vi "Dashboard Main.vi"() -> ()   [LabVIEW 2015]
uses:
  <vilib>/Utility/miscctls.llb/LVRowAndColumnTypeDef.ctl
  <vilib>/event_ctls.llb/eventvkey.ctl
  <vilib>/Rock Robotics/WPI/Dashboard/WPI_DashboardLogging Global.vi
  <vilib>/Utility/config.llb/Write Key (String).vi
  <vilib>/Utility/config.llb/Write Key (I32).vi
  <vilib>/Utility/config.llb/NI_LVConfig.lvlib
panel:
  in  "TCP":refnum<k5>
  in  "Rec Mode":enum32{"Stop", "Record", "Playback"}(radio)
  in  "Vision":u16(ring) items=["Camera Off", "USB Camera SW", "USB Camera HW", "IP Camera"]
  out "Camera IP":string
  out "Image Message":string="Timeout in Camera Communications"
  in  "Dashboard Tab":T1(tab)
  in  "Auto":string(combo)
  out "Velocity":dbl
  out "Can Hit":bool
  out "Visible Image":bool
  out "Can Hit":bool
  out "Possible Velocity":bool
  out "Centered":bool
  in  "Select Auto":string(combo)
  out "NT Connection":bool
  in  "Camera Settings":T2={"Frame Rate"=30, "Compression"=30, "Size"=1} {"Frame Rate" scale=1.0..30.0; "Size" items=["640x480", "320x240", "160x120"]}
  out "Mode":T3(ring)=enum."Auto Disabled"
  in  "DB Camera Config":bool
  out "fps":dbl format="%#.1g"
  out "Mbps":dbl format="%#.1g"
  out "Mbps LED":bool
  in  "DB/String 9":string
  in  "DB/String 8":string
  in  "DB/String 7":string
  in  "DB/String 6":string
  in  "DB/String 5":string
  in  "DB/String 4":string
  in  "DB/String 3":string
  in  "DB/String 2":string
  in  "DB/String 1":string
  in  "DB/String 0":string
  in  "DB/Slider 0":dbl(slide) scale=0.0..5.0
  in  "DB/Slider 1":dbl(slide) scale=0.0..5.0
  in  "DB/Slider 2":dbl(slide) scale=0.0..5.0
  in  "DB/Slider 3":dbl(slide) scale=0.0..5.0
  out "DB/LED 3":bool
  out "DB/LED 2":bool
  out "DB/LED 1":bool
  out "DB/LED 0":bool
  in  "DB/Button 3":bool
  in  "DB/Button 2":bool
  in  "DB/Button 1":bool
  in  "DB/Button 0":bool caption="New Name"
  in  "Test Slider":dbl(slide) scale=0.0..100.0 scale format="%#_3g"
  in  "On/Off":bool caption="Solenoid"
  in  "Test Name":u16(ring) items=["Select the test to run..."]
  in  "Test Tree":string(tree)
  in  "Motor":cluster{"Value":dbl, "Enable":bool} {"Value" scale=-1.0..1.0 scale format="%#_3g"}
  out "Progress":T4 {"Test Progress" scale=0.0..100.0}
  in  "Rev/Fwd":cluster{"Forward":bool, "Reverse":bool}
  in  "Test Ring":u16(ring) items=["Monochrome", "Color"]
  out "Cmd Status":string
  in  "Execute Command":bool
  in  "Command Params":string[][](table)
  in  "Command Selection":i32(listbox)
  in  "CheckList":i32(listbox)
  out "Tree":string(tree)
  out "Camera Image":T5(plugin-control)
  out "Background":bool
  # "This tab is a great place for autonomous settings and robot-specific values.\nPlace controls and indicators inside this tab and match name to\nDashboard Variables on robot. You can also delete this comment."
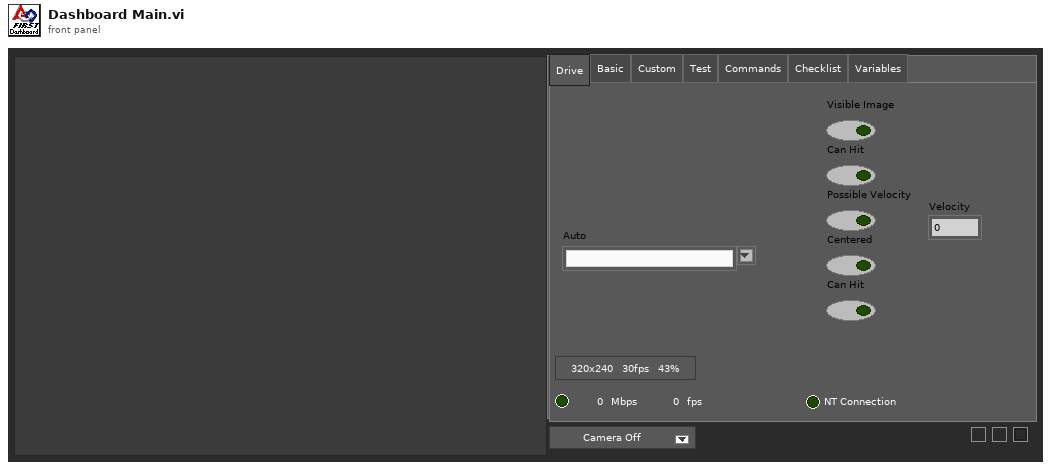
[diagram p1: front panel]
types:
  T1 = enum32{"Drive", "Basic", "Custom", "Test", "Commands", "Checklist", "Variables"}
  T2 = cluster{"Frame Rate":i32, "Compression":i32, "Size":u16}
  T3 = enum8{"Tele-Op Disabled", "Tele-Op Enabled", "Auto Disabled", "Auto Enabled", "Test Disabled", "Test Enabled", "Disconnected", "No Code", "E-Stop"}
  T4 = cluster{"Test Progress":u8, "Test Progress Text":string}
  T5 = typedef "IMAQ Image.ctl" = refnum<image>
  T6 = cluster{"IDs":cluster{"RPC field ID":u16, "Unique ID":u16}, "String":string}
  T7 = enum32{"Drive", "Basic", "Custom", "Test", "Checklist", "Variables"}
  T8 = typedef "Image Type" = u32
  T9 = cluster{"Camera Image":refnum<vi>, "Dashboard Tab":refnum<vi>, "Background":refnum<vi>, "Vision":refnum<vi>, "Rec Mode":refnum<vi>, "Test Slider":refnum<vi>, "On/Off ":refnum<vi>, "Test Ring":refnum<vi>, "Rev/Fwd":refnum<vi>, "Test Name":refnum<vi>, "Motor":refnum<vi>, "Progress":refnum<vi>, "CheckList":refnum<vi>, "Tree":refnum<vi>, "Test Tree":refnum<vi>, "Command Params":refnum<vi>, "Command Selection":refnum<vi>, "Execute Command":refnum<vi>, "Cmd Status":refnum<vi>}
  T10 = cluster{"Error Strings":string, "Disable Counts":cluster{u16, u16}, "Rail Faults":cluster{u16, u16, u16}, "Robot IP":string, "DB Mode":u8, "Event Info":cluster{"Name":string, "Type":u8, "Number":u16, "Replay":u8}, "Camera Addr":string}
  T11 = cluster{"Storage":cluster{"Disk Free":u64, "RAM Block":u32, "RAM free":u32}, "CPU Utilization":cluster{"CPU % ISR":sgl, "CPU % Time Crit":sgl, "CPU % Timed Str":sgl, "CPU % High":sgl, "CPU % Above":sgl, "CPU % Normal":sgl, "CPU % Low":sgl}, "CAN":cluster{"% Bus Utilization":sgl, "Bus Off Cnt":u32, "TX_FIFO Full Cnt":u32, "Receive Error Cnt":u8, "Transmit Error Cnt":u8}, "HID":cluster{"HID Outputs":u32, "Rumble Low":u16, "Rumble High":u16}[]}
  T12 = cluster{"Status bits":cluster{"Test Mode":bool, "Autonomous":bool, "Enabled":bool, "Code Start":bool, "Brownout":bool, "Reserved 2":bool, "Reserved 3":bool, "E-Stop":bool}, "Code Trace":cluster{"Disabled":bool, "TeleOp":bool, "Auto":bool, "Test":bool}, "Controller Type":enum16{"unknown", "cRIO", "roboRio"}, "Code?":enum16{"unknown", "noCode", "code"}, "Battery V":dbl}
  T13 = cluster{"Control Bits":cluster{"TestMode":bool, "Autonomous":bool, "Enabled":bool, "FMS Present":bool, bool, bool, bool, "E-Stop":bool}, "Team Station ":u8, "Countdown":sgl, "Joystick Values":cluster{"Axes":dbl[], "Buttons":bool[], "POVs":i16[]}[]}
  T14 = typedef "NI_LVConfig.lvlib/Config Data RefNum.ctl" = refnum<k1>
  T15 = cluster{"Operation":enum16{"Update", "Clear"}, "Color Box":u32}[]
  T16 = typedef "eventvkey.ctl" = enum16{"ASCII", "Enter", "Return", "Shift", "Ctrl", "Alt", "Cmd", "Opt", "Caps", "NumLock", "Clear", "Break", "Up", "Down", "Left", "Right", "Insert", "Delete", "Home", "End", "PageUp", "PageDown", "Escape", "Help", "Pause", "ScrollLock", "F1", "F2", "F3", "F4", "F5", "F6", "F7", "F8", "F9", "F10", "F11", "F12", "F13", "F14", "F15", "F16", "F17", "F18", "F19", "F20", "F21", "F22", "F23", "F24", "Play", "VolumeUp", "VolumeDown", "Mute", "Two Byte Char"}
  T17 = cluster{"Image Size":bool, "Image Type":bool, "Pixel Value":bool, "ROI Information":bool, "Zoom Factor":bool}
  T18 = enum8{"Enabled", "Disabled", "Disabled and Grayed Out"}
  T19 = cluster{"Operation":enum16{"Update", "Clear"}, "Color Box":u32}
  T20 = typedef "LVRowAndColumnTypeDef.ctl" = cluster{"Row":i32, "Column":i32}
  T21 = cluster{"Shift":bool, "Ctrl":bool, "Alt":bool, "Cmd":bool, "Opt":bool}
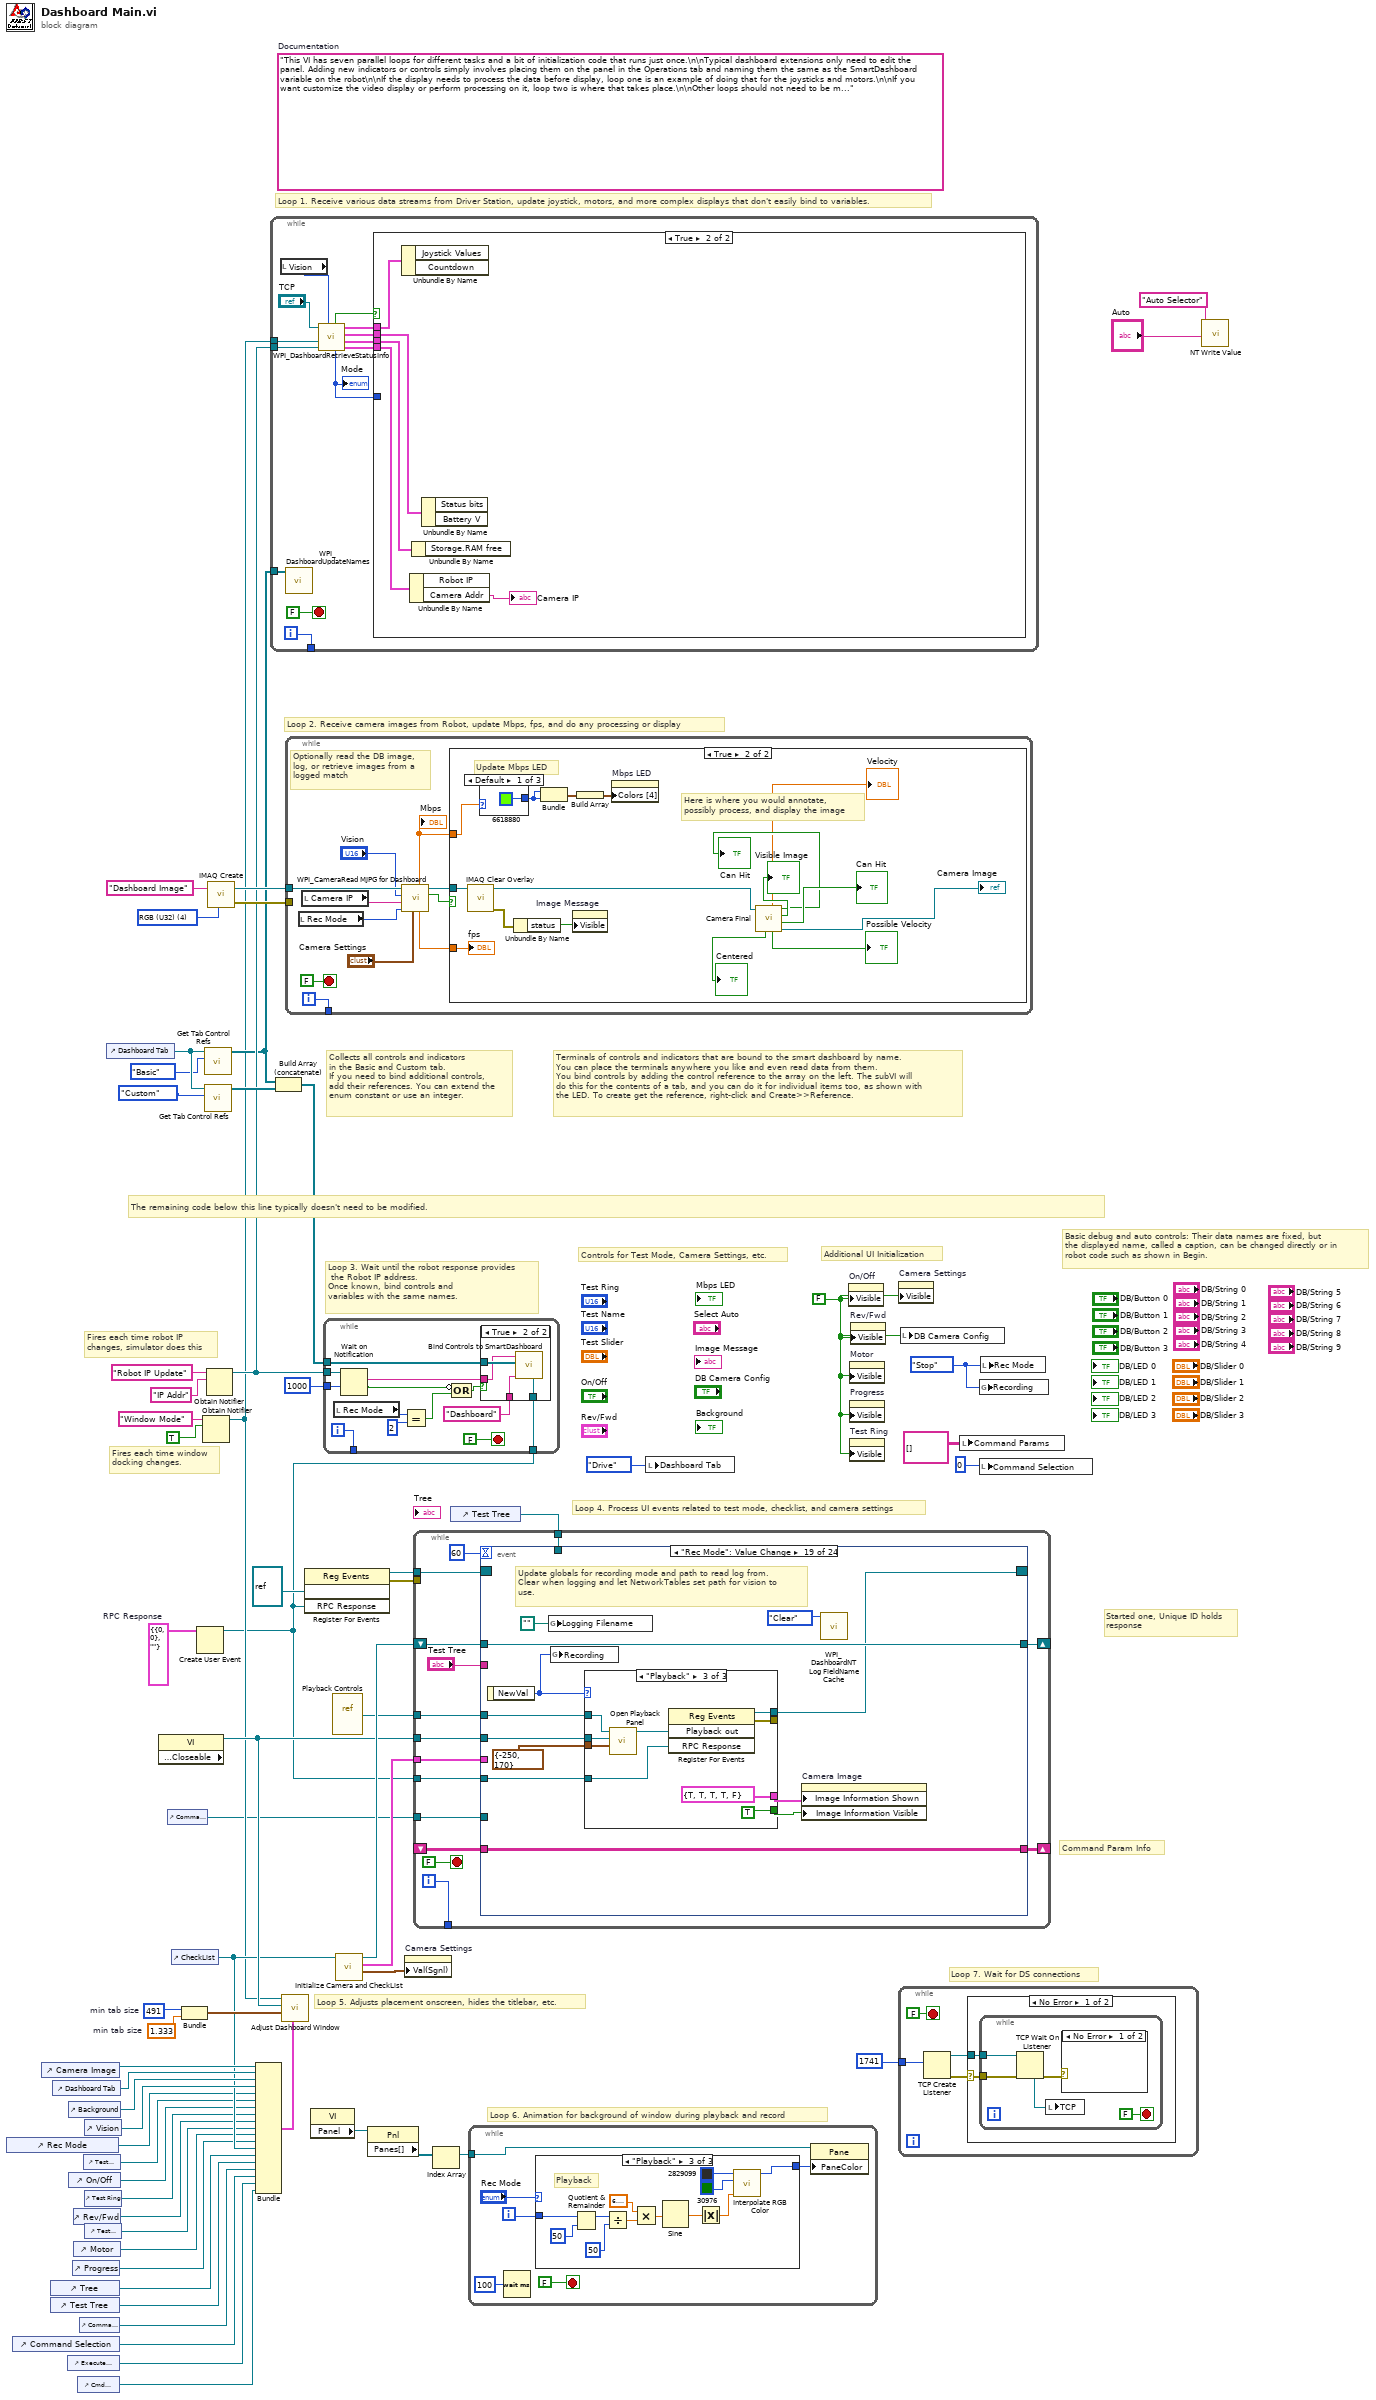
[diagram p0: block diagram]
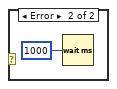
[diagram p2: hidden frame]
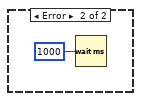
[diagram p3: hidden frame]
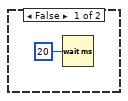
[diagram p4: hidden frame]
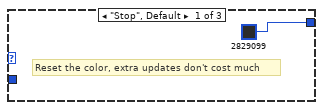
[diagram p5: hidden frame]
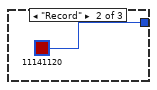
[diagram p6: hidden frame]
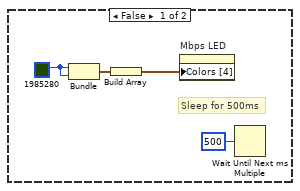
[diagram p8: hidden frame]
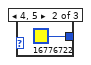
[diagram p9: hidden frame]
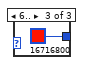
[diagram p10: hidden frame]
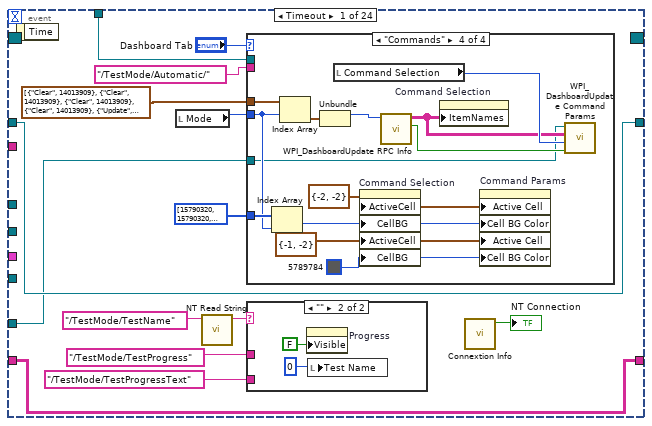
[diagram p11: hidden frame]
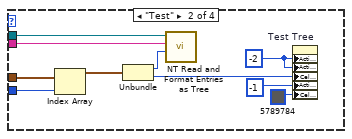
[diagram p13: hidden frame]
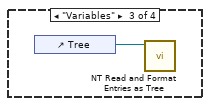
[diagram p14: hidden frame]
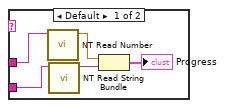
[diagram p15: hidden frame]
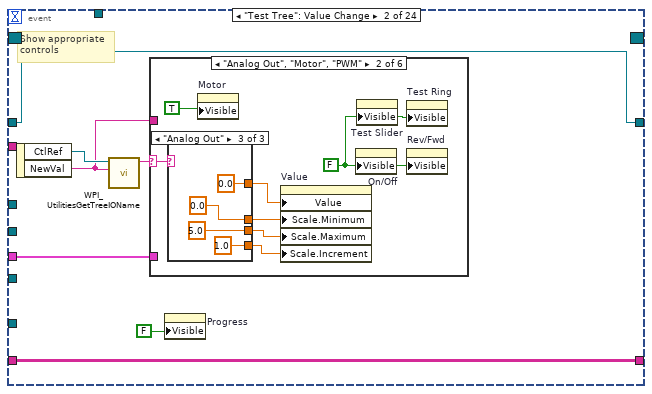
[diagram p16: hidden frame]
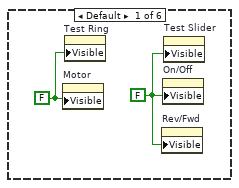
[diagram p17: hidden frame]
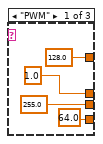
[diagram p18: hidden frame]
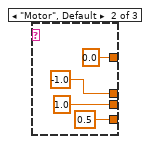
[diagram p19: hidden frame]
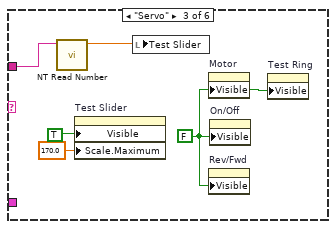
[diagram p20: hidden frame]
diagram:
  w9 = T6 {"IDs"={"RPC field ID"=0, "Unique ID"=0}, "String"=""}  # RPC Response
  w35 = 491  # min tab size
  w34 = 1.333  # min tab size
  w43 = enum32{"Stop", "Record", "Playback"}."Stop" ("Rec Mode")
  w17 = FALSE ("Visible")
  (unwired) "This VI has seven parallel loops for different tasks and a bit of initialization code that runs just once.\n\nTypical dashboard extensions only need to edit the panel. Adding new indicators or controls simply involves placing them on the panel in the Operations tab and naming them the same as the SmartDashboard variable on the robot\n\nIf the display needs to process the data before display, loop one is an example of doing that for the joysticks and motors.\n\nIf you want customize the video display or perform processing on it, loop two is where that takes place.\n\nOther loops should not need to be modified. They are pretty standard, and document the task they perform."  # Documentation
  w63 = T8 4 items=["Grayscale (U8)", "Grayscale (I16)", "Grayscale (SGL)", "Complex (CSG)", "RGB (U32)", "HSL (U32)", "RGB (U64)"] ("Image Type")
  # "Command Param Info"
  # "Started one, Unique ID holds\nresponse"
  # "Loop 7. Wait for DS connections"
  # "Basic debug and auto controls: Their data names are fixed, but\nthe displayed name, called a caption, can be changed directly or in\nrobot code such as shown in Begin."
  # "Controls for Test Mode, Camera Settings, etc."
  # "Additional UI Initialization"
  # "Loop 6. Animation for background of window during playback and record"
  # "Fires each time robot IP\nchanges, simulator does this"
  # "Fires each time window\ndocking changes."
  # "Collects all controls and indicators\nin the Basic and Custom tab.\nIf you need to bind additional controls,\nadd their references. You can extend the\nenum constant or use an integer."
  # "The remaining code below this line typically doesn't need to be modified."
  # "Loop 4. Process UI events related to test mode, checklist, and camera settings"
  # "Terminals of controls and indicators that are bound to the smart dashboard by name.\nYou can place the terminals anywhere you like and even read data from them.\nYou bind controls by adding the control reference to the array on the left. The subVI will\ndo this for the contents of a tab, and you can do it for individual items too, as shown with\nthe LED. To create get the reference, right-click and Create>>Reference."
  # "Loop 3. Wait until the robot response provides\n the Robot IP address.\nOnce known, bind controls and\nvariables with the same names."
  # "Loop 5. Adjusts placement onscreen, hides the titlebar, etc."
  # "Loop 1. Receive various data streams from Driver Station, update joystick, motors, and more complex displays that don't easily bind to variables."
  # "Loop 2. Receive camera images from Robot, update Mbps, fps, and do any processing or display"
  n1 = control-ref of="Rec Mode"() -> (w23:refnum<vi>)
  n2 = control-ref of="Command Selection"() -> (w8:refnum<vi>)
  n3 = control-ref of="Camera Image"() -> (w38:refnum<vi>)
  n4 = control-ref of="Tree"() -> (w27:refnum<vi>)
  n5 = control-ref of="Test Tree"() -> (w26:refnum<vi>)
  n6 = control-ref of="Dashboard Tab"() -> (w37:refnum<vi>)
  n7 = control-ref of="Execute Command"() -> (w10:refnum<vi>)
  n8 = control-ref of="Background"() -> (w32:refnum<vi>)
  n9 = control-ref of="On/Off"() -> (w21:refnum<vi>)
  n10 = control-ref of="Progress"() -> (w18:refnum<vi>)
  n11 = control-ref of="Rev/Fwd"() -> (w19:refnum<vi>)
  n12 = control-ref of="Motor"() -> (w24:refnum<vi>)
  n13 = control-ref of="Cmd Status"() -> (w4:refnum<vi>)
  n14 = control-ref of="Command Params"() -> (w11:refnum<vi>)
  n15 = control-ref of="Test Slider"() -> (w22:refnum<vi>)
  n16 = control-ref of="Vision"() -> (w36:refnum<vi>)
  n17 = control-ref of="Test Ring"() -> (w20:refnum<vi>)
  n18 = control-ref of="Test Name"() -> (w25:refnum<vi>)
  n19 = control-ref of="Dashboard Tab"() -> (w41:refnum<vi>)
  n20 = property class="VI" props=["Front Panel.Closeable"]() -> (reference out=w42:refnum<vi>)  [unwired: 2 in, 2 out]
  n21 = control-ref of="Command Params"() -> (w3:refnum<vi>)
  n22 = control-ref of="CheckList"() -> (w28:refnum<vi>)
  n23 = Bundle("min tab size"=w35, "min tab size"=w34) -> (w33:cluster{"min tab size":i32, "min tab size":dbl})  [unwired: 1 in]
  n24 = Create User Event(user event datatype=w9) -> (user event=w5:refnum<user-event>)  [unwired: 1 in, 1 out]
  n25 = Obtain Notifier(name (unnamed)="Window Mode", notification data type=TRUE) -> (notifier out=w14:refnum<notifier>)  [unwired: 2 in, 2 out]
  n26 = call <vilib>:"Get Tab Control Refs.vi"("Page Index"=T7."Basic" ("Dashboard Tab"), "TabControl in"=w41) -> ("ControlsOnPage"=w15:refnum<vi>[])  [unwired: 9 in]
  n27 = call <vilib>:"Get Tab Control Refs.vi"("Page Index"=T7."Custom" ("Dashboard Tab"), "TabControl in"=w41) -> ("ControlsOnPage"=w40:refnum<vi>[])  [unwired: 9 in]
  n28 = Obtain Notifier(name (unnamed)="Robot IP Update", notification data type="IP Addr" ("name (unnamed)")) -> (notifier out=w16:refnum<notifier>)  [unwired: 2 in, 2 out]
  n29 = call "IMAQ Create"("Image Name"="Dashboard Image", "Image Type"=w63) -> ("New Image"=w61:T5, "error out"=w60:errorcluster)  [unwired: 2 in, 1 out]
  n30 = Bundle("Camera Image"=w38, "Dashboard Tab"=w37, "Background"=w32, "Vision"=w36, "Rec Mode"=w23, "Test Slider"=w22, "On/Off"=w21, "Test Ring"=w20, "Rev/Fwd"=w19, "Test Name"=w25, "Motor"=w24, "Progress"=w18, "CheckList"=w28, "Tree"=w27, "Test Tree"=w26, "Command Params"=w11, "Command Selection"=w8, "Execute Command"=w10, "Cmd Status"=w4) -> (w29:T9)  [unwired: 1 in]
  n31 = while {
    tunnel: [w75] -> _
    tunnel: w16 -> [w69]
    tunnel: w15 -> [w68]
    tunnel: w14 -> [w64]
    i -> [w75]
    stop <- FALSE stop-if-true
    n32 = local read "Vision"() -> (w66:u16)
    n33 = call <vilib>:"WPI_DashboardUpdateNames.vi"("Controls on Tab"=w68) -> ()  [unwired: 11 in]
    n34 = call <vilib>:"WPI_DashboardRetrieveStatusInfo.vi"("Vision"=w66, "Binding Refnum"=w69, "Window Mode Notifier"=w64, "TCP Cnx"="TCP") -> ("Power and Errors"=w70:T10, "Robot Metrics"=w73:T11, "Status Info"=w74:T12, "Control Info"=w71:T13, "Robot Mode"=w67:T3, "Process?"=w72:bool)  [unwired: 2 in]
    "Mode" <- w67
    n35 = case shown="True" w72 {
      tunnel: w74 -> [_ w82]
      tunnel: w73 -> [_ w81]
      tunnel: w71 -> [_ w80]
      tunnel: w70 -> [_ w79]
      tunnel: w67 -> [_ _]
      frame False {
        n36 = Wait (ms)(milliseconds to wait=u32 20) -> ()  [unwired: 1 out]
      }
      frame True {
        n37 = Unbundle By Name(w80) -> ()  [unwired: 2 out]
        n38 = Unbundle By Name(w79) -> ("Camera Addr"=→"Camera IP":string)  [unwired: 1 out]
        n39 = Unbundle By Name(w81) -> ()  [unwired: 1 out]
        n40 = Unbundle By Name(w82) -> ()  [unwired: 2 out]
      }
    }
  }
  n41 = Build Array (concatenate)(w15, w40) -> (w39:refnum<vi>[])
  n42 = call "Adjust Dashboard Window.vi"("Sizing Refnums"=w29, "Size Constraints"=w33, "VI"=w42, "WIn Mode"=w14) -> ()  [unwired: 8 in]
  n43 = while {
    tunnel: w61 -> [w91]
    tunnel: w60 -> [_]
    tunnel: [w92] -> _
    i -> [w92]
    stop <- FALSE stop-if-true
    # "Optionally read the DB image,\nlog, or retrieve images from a\nlogged match"
    n44 = local read "Rec Mode"() -> (w86:enum32{"Stop", "Record", "Playback"})
    n45 = local read "Camera IP"() -> (w84:string)
    n46 = call <vilib>:"WPI_CameraRead MJPG for Dashboard.vi"("Camera Settings"="Camera Settings", "Rec Mode"=w86, "Camera IP"=w84, "Camera Mode"="Vision", "Refnum in"=w91) -> ("Active"=w89:bool, "Refnum out"=w90:T5, "FPS"=w88:dbl, "Bandwidth (Mbps)"=w83:dbl)  [unwired: 3 in]
    "Mbps" <- w83
    n47 = case shown="True" w89 {
      tunnel: w90 -> [_ w108]
      tunnel: w83 -> [_ w107]
      tunnel: w88 -> [_ w106]
      frame False {
        w94 = u32 1985280 ("Color Box")
        # "Sleep for 500ms"
        n48 = Bundle("Color Box"=w94, "Color Box"=w94) -> (w96:cluster{"Color Box":u32, "Color Box":u32})  [unwired: 1 out]
        n49 = Build Array(w96) -> (w95:cluster{"Color Box":u32, "Color Box":u32}[])
        n50 = property on="Mbps LED" class="Bool (strict)"("Colors [4]"=w95) -> ()  [unwired: 2 in, 2 out]
        n51 = Wait Until Next ms Multiple(millisecond multiple=u32 500) -> ()  [unwired: 1 out]
      }
      frame True {
        # "Here is where you would annotate,\npossibly process, and display the image"
        # "Update Mbps LED"
        n52 = call "IMAQ Clear Overlay"("Image"=w108) -> ("error out"=w112:errorcluster, "Image Out"=w105:T5)  [unwired: 2 in, 7 out]
        n53 = case shown="Default" w107 {
          tunnel: [u32 6618880 ("Color Box") u32 16776722 ("Color Box") u32 16716800 ("Color Box")] -> w109
          frame Default {
          }
          frame 4, 5 {
          }
          frame 6.. {
          }
        }
        n54 = Unbundle By Name(w112) -> ("status"=w113:bool)
        n55 = Bundle("Color Box"=w109, "Color Box"=w109) -> (w111:cluster{"Color Box":u32, "Color Box":u32})  [unwired: 1 out]
        n56 = property on="Image Message" class="Str"("Visible"=w113) -> ()  [unwired: 2 in, 2 out]
        n57 = Build Array(w111) -> (w110:cluster{"Color Box":u32, "Color Box":u32}[])
        n58 = property on="Mbps LED" class="Bool (strict)"("Colors [4]"=w110) -> ()  [unwired: 2 in, 2 out]
        n59 = call "Camera Final.vi"("Image Src"=w105) -> ("Image Dst Out 2"=→"Camera Image":T5, "Can Fit"=→"Can Hit":bool, "Viable Image"=→"Visible Image":bool, "Can Hit"=→"Can Hit":bool, "Possible Velocity"=→"Possible Velocity":bool, "Velocity"=→"Velocity":dbl, "Centered"=→"Centered":bool)  [unwired: 4 in]
        "fps" <- w106
      }
    }
  }
  n60 = register-events(refnum<vi> refnum, w5) -> (reference out=w47:refnum<event-registration>, error out=w46:errorcluster)  [unwired: 2 in]
  n61 = property class="VI"() -> ("Panel"=w50:refnum<vi>)  [unwired: 2 in, 2 out]
  n62 = while {
    tunnel: w39 -> [w129]
    tunnel: w16 -> [w127]
    tunnel: [w125] -> _
    tunnel: u32 1000 ("milliseconds to wait") -> [w124]
    tunnel: w5 -> [w117]
    i -> [w125]
    stop <- FALSE stop-if-true
    n63 = local read "Rec Mode"() -> (w120:enum32{"Stop", "Record", "Playback"})
    n64 = Wait on Notification(notifier=w127, timeout in ms (-1)=w124) -> (notification=w126:string, timed out?=w122:bool)  [unwired: 2 in, 2 out]
    n65 = Equal?(x=w120, y=u16 2 ("Rec Mode")) -> (x = y?=w121:bool)
    n66 = Compound Arithmetic op=OR(invert w122, w121) -> (w123:bool)
    n67 = case shown="True" w123 {
      tunnel: w129 -> [_ w133]
      tunnel: w126 -> [_ w132]
      tunnel: "Dashboard" -> [_ w131]
      tunnel: w117 -> [_ w130]
      frame False {
      }
      frame True {
        n68 = call <vilib>:"Bind Controls to SmartDashboard.vi"("RPC ref"=w130, "Client Name"=w131, "Bound Control Refs"=w133, "Server IP Address"=w132) -> ()  [unwired: 8 in]
      }
    }
  }
  n69 = vi-ref "Playback Controls.vi"() -> (w48:refnum<vi>)
  n70 = call "Initialize Camera and CheckList.vi"("ListBox in"=w28) -> ("Cluster"=w54:cluster{"value":i32, "value":i32, "index":i32}, "Array"=w55:cluster{string[]}[], "File Refnum"=w53:T14)  [unwired: 8 in]
  n71 = property class="Pnl"(reference=w50) -> ("Panes[]"=w51:refnum<vi>[])  [unwired: 1 in, 2 out]
  n72 = property on="Camera Settings" class="Clust (strict)"("Val(Sgnl)"=w54) -> ()  [unwired: 2 in, 2 out]
  n73 = Index Array(array=w51) -> (element=w49:refnum<vi>)  [unwired: 1 in]
  n74 = control-ref of="Test Tree"() -> (w52:refnum<vi>)
  n75 = while {
    tunnel: w55 -> [w145]
    shift-right: [w144] -> _
    shift-left: w53 -> [w143]
    tunnel: [w142] -> _
    tunnel: w52 -> [w141]
    tunnel: w48 -> [w140]
    tunnel: w47 -> [w139]
    tunnel: w46 -> [_]
    tunnel: w42 -> [w138]
    tunnel: w5 -> [w137]
    tunnel: w3 -> [w136]
    shift-right: [w135] -> _
    shift-left: _ -> [w134]
    i -> [w142]
    stop <- FALSE stop-if-true
    n76 = event shown="[18] \"Rec Mode\": Value Change" {
      selector: w139 -> [_ _ _ _ _ _ _ _ _ _ _ _ _ _ _ _ _ _ _ _ _ _ _ _]
      dyn-events: [_ _ _ _ _ _ _ _ _ _ _ _ _ _ _ _ _ _ w454 _ _ _ _ _] -> _
      timeout: u32 60 ("milliseconds to wait") -> [_ _ _ _ _ _ _ _ _ _ _ _ _ _ _ _ _ _ _ _ _ _ _ _]
      tunnel: w141 -> [w159 _ _ _ _ _ _ _ _ _ _ _ _ _ _ _ _ _ _ _ _ _ _ _]
      tunnel: "Test Tree" -> [_ _ _ _ _ _ _ _ _ _ _ _ _ w417 w426 w429 w434 w443 _ _ _ _ _ _]
      tunnel: w145 -> [_ w196 _ _ _ _ _ _ _ _ _ w379 w410 _ _ _ _ _ _ _ _ _ _ _]
      tunnel: [w156 w195 w299 w305 w315 w319 w325 w337 w345 w351 w364 w378 w403 w416 w424 w428 w433 w442 w456 w472 w474 w482 w493 w498] -> w144
      tunnel: w143 -> [w156 w195 w299 w305 w315 w319 w325 w337 w345 w351 w364 w377 w403 w416 w424 w428 w433 w442 w456 w472 w474 w482 w493 w498]
      tunnel: w140 -> [_ _ _ _ _ _ _ _ _ _ _ _ _ _ _ _ _ _ w457 _ w477 _ _ _]
      tunnel: w138 -> [_ _ _ _ _ _ _ _ _ _ _ _ _ _ _ _ _ _ w452 _ _ _ _ _]
      tunnel: w137 -> [_ _ _ _ _ _ _ _ _ _ _ _ _ _ _ _ _ _ w448 _ _ _ _ _]
      tunnel: w136 -> [w151 _ _ _ _ _ w323 _ _ _ _ _ _ _ _ _ _ _ _ _ _ _ _ _]
      tunnel: [w150 w194 w298 w304 w314 w320 w321 w331 w342 w350 w363 w376 w402 w415 w423 w427 w432 w441 w447 w470 w473 w478 w486 w499] -> w135
      tunnel: w134 -> [w150 w194 w298 w304 w314 w320 w321 _ _ w350 w363 w376 w402 w415 w423 w427 w432 w441 w447 w470 w473 w478 w486 w499]
      event Timeout {
        n77 = event-data() -> ()  [unwired: 1 in, 1 out]
        n78 = local read "Mode"() -> (w153:T3)
        n79 = call <vilib>:"NT Read String.vi"("Name"="/TestMode/TestName") -> ("String"=w161:string)  [unwired: 9 in, 1 out]
        n80 = case shown="\"Commands\"" "Dashboard Tab" {
          tunnel: w159 -> [_ w172 _ _]
          tunnel: "/TestMode/Automatic/" ("Name Pattern") -> [_ w171 _ _]
          tunnel: T15 [{"Operation"=enum."Clear", "Color Box"=14013909}, {"Operation"=enum."Clear", "Color Box"=14013909}, {"Operation"=enum."Clear", "Color Box"=14013909}, {"Operation"=enum."Clear", "Color Box"=14013909}, {"Operation"=enum."Update", "Color Box"=14013909}, {"Operation"=enum."Update", "Color Box"=16777215}, {"Operation"=enum."Clear", "Color Box"=14013909}, {"Operation"=enum."Clear", "Color Box"=14013909}, {"Operation"=enum."Clear", "Color Box"=14013909}] -> [_ w164 _ w181]
          tunnel: w153 -> [_ w163 _ w180]
          tunnel: u32[] [15790320, 15790320, 15790320, 15790320, 16777215, 16777215, 15790320, 15790320, 15790320] -> [_ _ _ w186]
          tunnel: w151 -> [_ _ _ w174]
          frame "Custom", Default {
          }
          frame "Test" {
            w170 = -2 ("Active Item:Row Number")
            n81 = Index Array(array=w164, index=w163) -> (element=w165:T19)
            n82 = Unbundle(w165) -> ("Operation"=w166:enum16{"Update", "Clear"}, "Color Box"=w167:u32)
            n83 = call <vilib>:"NT Read and Format Entries as Tree.vi"("Operation"=w166, "Name Pattern"=w171, "Tree Refnum"=w172) -> ()  [unwired: 7 in, 2 out]
            n84 = property on="Test Tree" class="Tree (strict)"("Active Item Row Number"=w170, "ActiveColNum"=w170, "CellBG"=w167, "Active Item Row Number"=-1 ("Active Item:Row Number"), "CellBG"=u32 5789784 ("Color Box")) -> ()  [unwired: 2 in, 2 out]
          }
          frame "Variables" {
            n85 = control-ref of="Tree"() -> (w173:refnum<vi>)
            n86 = call <vilib>:"NT Read and Format Entries as Tree.vi"("Tree Refnum"=w173) -> ()  [unwired: 9 in, 2 out]
          }
          frame "Commands" {
            w182 = u32 5789784 ("Color Box")
            w183 = T20 {"Row"=-1, "Column"=-2} ("Active Cell:Active Cell")
            w185 = T20 {"Row"=-2, "Column"=-2} ("Active Cell:Active Cell")
            n87 = Index Array(array=w186, index=w180) -> (element=w184:u32)
            n88 = Index Array(array=w181, index=w180) -> (element=w179:T19)
            n89 = Unbundle(w179) -> ("Operation"=w178:enum16{"Update", "Clear"})  [unwired: 1 out]
            n90 = local read "Command Selection"() -> (w177:i32)
            n91 = property on="Command Selection" class="MCListbox (strict)"("ActiveCell"=w185, "CellBG"=w184, "ActiveCell"=w183, "CellBG"=w182) -> ()  [unwired: 2 in, 2 out]
            n92 = call <vilib>:"WPI_DashboardUpdate RPC Info.vi"("Operation"=w178) -> ("update"=w176:bool, "commands"=w175:string[][])  [unwired: 9 in]
            n93 = property on="Command Selection" class="MCListbox (strict)"("ItemNames"=w175) -> ()  [unwired: 2 in, 2 out]
            n94 = property on="Command Params" class="Tbl (strict)"("Active Cell"=w185, "Cell BG Color"=w184, "Active Cell"=w183, "Cell BG Color"=w182) -> ()  [unwired: 2 in, 2 out]
            n95 = call <vilib>:"WPI_DashboardUpdate Command Params.vi"("Update"=w176, "NewVal"=w177, "Commands"=w175, "Param Tbl"=w174) -> ()  [unwired: 7 in, 1 out]
          }
        }
        n96 = case shown="\"\"" w161 {
          tunnel: "/TestMode/TestProgress" ("Name") -> [w188 _]
          tunnel: "/TestMode/TestProgressText" ("Name") -> [w187 _]
          frame Default {
            n97 = call <vilib>:"NT Read Number.vi"("Name"=w188) -> ("Numeric"=w189:dbl)  [unwired: 9 in, 1 out]
            n98 = call <vilib>:"NT Read String.vi"("Name"=w187) -> ("String"=w190:string)  [unwired: 9 in, 1 out]
            n99 = Bundle("Numeric"=w189, "String"=w190) -> (→"Progress":cluster{"Numeric":dbl, "String":string})  [unwired: 1 in]
          }
          frame "" {
            n100 = property on="Progress" class="Clust (strict)"("Visible"=FALSE) -> ()  [unwired: 2 in, 2 out]
            n101 = local write "Test Name"(u16 0) -> ()
          }
        }
        n102 = call <vilib>:"Connextion Info.vi"() -> ("Connected"=→"NT Connection":bool)  [unwired: 10 in, 1 out]
      }
      event "Test Tree": Value Change {
        # "Show appropriate\ncontrols"
        n103 = event-data() -> ("CtlRef"=w199:refnum<vi>, "NewVal"=w197:string)  [unwired: 1 in]
        n104 = call <vilib>:"WPI_UtilitiesGetTreeIOName.vi"("NewVal"=w197, "TreeControl in"=w199) -> ("I/O Name"=w200:string)  [unwired: 9 in]
        n105 = case shown="\"Analog Out\", \"Motor\", \"PWM\"" w200 {
          selector: w200 -> [_ w207 _ w229 w238 _]
          tunnel: w197 -> [_ _ w226 w228 _ w245]
          tunnel: w196 -> [_ _ _ _ _ w244]
          frame Default {
            w202 = FALSE ("Visible")
            w201 = FALSE ("Visible")
            n106 = property on="Motor" class="Clust (strict)"("Visible"=w201) -> ()  [unwired: 2 in, 2 out]
            n107 = property on="Test Ring" class="Ring (strict)"("Visible"=w201) -> ()  [unwired: 2 in, 2 out]
            n108 = property on="Rev/Fwd" class="Clust (strict)"("Visible"=w202) -> ()  [unwired: 2 in, 2 out]
            n109 = property on="On/Off" class="Bool (strict)"("Visible"=w202) -> ()  [unwired: 2 in, 2 out]
            n110 = property on="Test Slider" class="Slide (strict)"("Visible"=w202) -> ()  [unwired: 2 in, 2 out]
          }
          frame "Analog Out", "Motor", "PWM" {
            w208 = FALSE ("Visible")
            n111 = case shown="\"Analog Out\"" w207 {
              tunnel: [1.0 ("Value") -1.0 ("Value") 0.0 ("Value")] -> w206
              tunnel: [255.0 ("Value") 1.0 ("Value") 5.0 ("Value")] -> w205
              tunnel: [128.0 ("Value") 0.0 ("Value") 0.0 ("Value")] -> w204
              tunnel: [64.0 ("Value") 0.5 ("Value") 1.0 ("Value")] -> w203
              frame "PWM" {
              }
              frame "Motor", Default {
              }
              frame "Analog Out" {
              }
            }
            n112 = property on="Motor" class="Clust (strict)"("Visible"=TRUE) -> ()  [unwired: 2 in, 2 out]
            n113 = property on="Value" class="Slide (strict)"("Value"=w204, "Scale.Minimum"=w206, "Scale.Maximum"=w205, "Scale.Increment"=w203) -> ()  [unwired: 2 in, 2 out]
            n114 = property on="On/Off" class="Bool (strict)"("Visible"=w208) -> ()  [unwired: 2 in, 2 out]
            n115 = property on="Test Slider" class="Slide (strict)"("Visible"=w208) -> ()  [unwired: 2 in, 2 out]
            n116 = property on="Test Ring" class="Ring (strict)"("Visible"=w208) -> ()  [unwired: 2 in, 2 out]
            n117 = property on="Rev/Fwd" class="Clust (strict)"("Visible"=w208) -> ()  [unwired: 2 in, 2 out]
          }
          frame "Servo" {
            w224 = FALSE ("Visible")
            n118 = call <vilib>:"NT Read Number.vi"("Name"=w226) -> ("Numeric"=w225:dbl)  [unwired: 9 in, 1 out]
            n119 = property on="Test Slider" class="Slide (strict)"("Visible"=TRUE, "Scale.Maximum"=170.0 ("Scale.Range:Maximum")) -> ()  [unwired: 2 in, 2 out]
            n120 = local write "Test Slider"(w225) -> ()
            n121 = property on="Motor" class="Clust (strict)"("Visible"=w224) -> ()  [unwired: 2 in, 2 out]
            n122 = property on="Rev/Fwd" class="Clust (strict)"("Visible"=w224) -> ()  [unwired: 2 in, 2 out]
            n123 = property on="On/Off" class="Bool (strict)"("Visible"=w224) -> ()  [unwired: 2 in, 2 out]
            n124 = property on="Test Ring" class="Ring (strict)"("Visible"=w224) -> ()  [unwired: 2 in, 2 out]
          }
          frame "Relay", "Solenoid" {
            w227 = FALSE ("Visible")
            n125 = property on="Motor" class="Clust (strict)"("Visible"=w227) -> ()  [unwired: 2 in, 2 out]
            n126 = property on="Test Slider" class="Slide (strict)"("Visible"=w227) -> ()  [unwired: 2 in, 2 out]
            n127 = Search and Replace String(input string=w228, search string="/Value  **", replace string="/Direction") -> (result string=w234:string)  [unwired: 5 in, 3 out]
            n128 = property on="Test Ring" class="Ring (strict)"("Visible"=w227) -> ()  [unwired: 2 in, 2 out]
            n129 = call <vilib>:"NT Read String.vi"("Name"=w234) -> ("String"=w232:string)  [unwired: 9 in, 1 out]
            n130 = Equal?(x="Both directions", y=w232) -> (x = y?=w230:bool)
            n131 = Not(x=w230) -> (.not. x?=w231:bool)
            n132 = property on="Rev/Fwd" class="Clust (strict)"("Visible"=w230) -> ()  [unwired: 2 in, 2 out]
            n133 = property on="On/Off" class="Bool (strict)"("Visible"=w231, "Caption.Text"=w229) -> ()  [unwired: 2 in, 2 out]
          }
          frame "Compressor", "Digital Out" {
            w237 = FALSE ("Visible")
            # "Get direction and finish"
            n134 = property on="Motor" class="Clust (strict)"("Visible"=w237) -> ()  [unwired: 2 in, 2 out]
            n135 = property on="Test Slider" class="Slide (strict)"("Visible"=w237) -> ()  [unwired: 2 in, 2 out]
            n136 = property on="Test Ring" class="Ring (strict)"("Visible"=w237) -> ()  [unwired: 2 in, 2 out]
            n137 = property on="On/Off" class="Bool (strict)"("Visible"=TRUE, "Caption.Text"=w238) -> ()  [unwired: 2 in, 2 out]
            n138 = property on="Rev/Fwd" class="Clust (strict)"("Visible"=FALSE) -> ()  [unwired: 2 in, 2 out]
          }
          frame "Camera" {
            n139 = call <vilib>:"Get Last Path Segment.vi"("String in"=w245) -> ("String out"=w246:string)  [unwired: 10 in]
            n140 = property on="On/Off" class="Bool (strict)"("Visible"=FALSE) -> ()  [unwired: 2 in, 2 out]
            n141 = property on="Motor" class="Clust (strict)"("Visible"=FALSE) -> ()  [unwired: 2 in, 2 out]
            n142 = property on="Rev/Fwd" class="Clust (strict)"("Visible"=FALSE) -> ()  [unwired: 2 in, 2 out]
            n143 = case shown="\"White Balance  **\"" w246 {
              tunnel: w245 -> [w252 w261 w270 w279 w288 _ w294]
              tunnel: w244 -> [w250 w258 w267 w276 w285 _ _]
              frame "Size  **" {
                n144 = Index Array(array=w250) -> (element=w249:cluster{string[]})  [unwired: 1 in]
                n145 = call <vilib>:"NT Read String.vi"("Name"=w252) -> ("String"=w251:string)  [unwired: 9 in, 1 out]
                n146 = Unbundle(w249) -> (w247:string[])
                n147 = Match First String(2:w247, 3:w251) -> (0:w248:i32)  [unwired: 1 out]
                n148 = property on="Test Ring" class="Ring (strict)"("Value"=w248, "Strings []"=w247) -> ()  [unwired: 2 in, 2 out]
                n149 = property on="Test Ring" class="Ring (strict)"("Visible"=TRUE) -> ()  [unwired: 2 in, 2 out]
                n150 = property on="Test Slider" class="Slide (strict)"("Visible"=FALSE) -> ()  [unwired: 2 in, 2 out]
              }
              frame "White Balance  **" {
                n151 = Index Array(array=w258, index=1) -> (element=w259:cluster{string[]})
                n152 = call <vilib>:"NT Read String.vi"("Name"=w261) -> ("String"=w260:string)  [unwired: 9 in, 1 out]
                n153 = Unbundle(w259) -> (w256:string[])
                n154 = Match First String(2:w256, 3:w260) -> (0:w255:i32)  [unwired: 1 out]
                n155 = property on="Test Ring" class="Ring (strict)"("Value"=w255, "Strings []"=w256) -> ()  [unwired: 2 in, 2 out]
                n156 = property on="Test Ring" class="Ring (strict)"("Visible"=TRUE) -> ()  [unwired: 2 in, 2 out]
                n157 = property on="Test Slider" class="Slide (strict)"("Visible"=FALSE) -> ()  [unwired: 2 in, 2 out]
              }
              frame "Exposure  **" {
                n158 = Index Array(array=w267, index=2) -> (element=w268:cluster{string[]})
                n159 = call <vilib>:"NT Read String.vi"("Name"=w270) -> ("String"=w269:string)  [unwired: 9 in, 1 out]
                n160 = Unbundle(w268) -> (w264:string[])
                n161 = Match First String(2:w264, 3:w269) -> (0:w265:i32)  [unwired: 1 out]
                n162 = property on="Test Ring" class="Ring (strict)"("Value"=w265, "Strings []"=w264) -> ()  [unwired: 2 in, 2 out]
                n163 = property on="Test Ring" class="Ring (strict)"("Visible"=TRUE) -> ()  [unwired: 2 in, 2 out]
                n164 = property on="Test Slider" class="Slide (strict)"("Visible"=FALSE) -> ()  [unwired: 2 in, 2 out]
              }
              frame "Exposure Priority  **" {
                n165 = Index Array(array=w276, index=3) -> (element=w277:cluster{string[]})
                n166 = call <vilib>:"NT Read String.vi"("Name"=w279) -> ("String"=w278:string)  [unwired: 9 in, 1 out]
                n167 = Unbundle(w277) -> (w273:string[])
                n168 = Match First String(2:w273, 3:w278) -> (0:w274:i32)  [unwired: 1 out]
                n169 = property on="Test Ring" class="Ring (strict)"("Value"=w274, "Strings []"=w273) -> ()  [unwired: 2 in, 2 out]
                n170 = property on="Test Ring" class="Ring (strict)"("Visible"=TRUE) -> ()  [unwired: 2 in, 2 out]
                n171 = property on="Test Slider" class="Slide (strict)"("Visible"=FALSE) -> ()  [unwired: 2 in, 2 out]
              }
              frame "Color Enable  **" {
                n172 = Index Array(array=w285, index=4) -> (element=w286:cluster{string[]})
                n173 = call <vilib>:"NT Read String.vi"("Name"=w288) -> ("String"=w287:string)  [unwired: 9 in, 1 out]
                n174 = Unbundle(w286) -> (w282:string[])
                n175 = Match First String(2:w282, 3:w287) -> (0:w283:i32)  [unwired: 1 out]
                n176 = property on="Test Ring" class="Ring (strict)"("Value"=w283, "Strings []"=w282) -> ()  [unwired: 2 in, 2 out]
                n177 = property on="Test Ring" class="Ring (strict)"("Visible"=TRUE) -> ()  [unwired: 2 in, 2 out]
                n178 = property on="Test Slider" class="Slide (strict)"("Visible"=FALSE) -> ()  [unwired: 2 in, 2 out]
              }
              frame Default {
                n179 = property on="Test Ring" class="Ring (strict)"("Visible"=FALSE) -> ()  [unwired: 2 in, 2 out]
                n180 = property on="Test Slider" class="Slide (strict)"("Visible"=FALSE) -> ()  [unwired: 2 in, 2 out]
              }
              frame "Brightness  **", "Color Level  **", "Compression  **", "FPS  **", "Sharpness  **" {
                n181 = call <vilib>:"NT Read Number.vi"("Name"=w294) -> ("Numeric"=w293:dbl)  [unwired: 9 in, 1 out]
                n182 = local write "Test Slider"(w293) -> ()
                n183 = property on="Test Slider" class="Slide (strict)"("Visible"=TRUE, "Scale.Maximum"=100.0 ("Scale.Range:Maximum")) -> ()  [unwired: 2 in, 2 out]
                n184 = property on="Test Ring" class="Ring (strict)"("Visible"=FALSE) -> ()  [unwired: 2 in, 2 out]
              }
            }
          }
        }
        n185 = property on="Progress" class="Clust (strict)"("Visible"=FALSE) -> ()  [unwired: 2 in, 2 out]
      }
      event "Test Name": Mouse Enter {
        # "Populate the ring with the list of tests"
        n186 = event-data() -> ()  [unwired: 1 in, 1 out]
        n187 = call <vilib>:"NT Read String Array.vi"("Name"="/TestMode/TestList") -> ("String Array"=w303:string[])  [unwired: 9 in, 1 out]
        n188 = Build Array (concatenate)("Select the test to run...", w303) -> (w302:string[])
        n189 = property on="Test Name" class="Ring (strict)"("Strings []"=w302) -> ()  [unwired: 2 in, 2 out]
      }
      event "Test Name": Value Change {
        w306 = FALSE ("Visible")
        # "Tell the robot the test name to run"
        n190 = event-data() -> ("NewVal"=w310:u16)  [unwired: 1 in]
        n191 = property on="Test Name" class="Ring (strict)"() -> ("Strings []"=w311:string[])  [unwired: 2 in, 2 out]
        n192 = local write "Progress"(T4 {"Test Progress"=0, "Test Progress Text"=""} ("Progress")) -> ()
        n193 = Index Array(array=w311, index=w310) -> (element=w309:string)
        n194 = call <vilib>:"NT Write String.vi"("String"=w309, "Name"="/TestMode/TestName") -> ()  [unwired: 9 in, 1 out]
        n195 = property on="Progress" class="Clust (strict)"("Visible"=TRUE) -> ()  [unwired: 2 in, 2 out]
        n196 = property on="Motor" class="Clust (strict)"("Visible"=w306) -> ()  [unwired: 2 in, 2 out]
        n197 = property on="Test Slider" class="Slide (strict)"("Visible"=w306) -> ()  [unwired: 2 in, 2 out]
        n198 = property on="On/Off" class="Bool (strict)"("Visible"=w306) -> ()  [unwired: 2 in, 2 out]
        n199 = property on="Rev/Fwd" class="Clust (strict)"("Visible"=w306) -> ()  [unwired: 2 in, 2 out]
        n200 = property on="Test Ring" class="Ring (strict)"("Visible"=w306) -> ()  [unwired: 2 in, 2 out]
      }
      event "Select Auto": Mouse Enter {
        # "Populate the combo box with the list of autonomous options"
        n201 = event-data() -> ()  [unwired: 1 in, 1 out]
        n202 = call <vilib>:"NT Read String Array.vi"("Name"="Auto List") -> ("String Array"=w313:string[])  [unwired: 9 in, 1 out]
        n203 = property on="Select Auto" class="CmbBox"("Strings[]"=w313) -> ()  [unwired: 2 in, 2 out]
      }
      event "Select Auto": Value Change {
        # "User modified the Auto Selection. Write to NT variable so robot knows."
        n204 = event-data() -> ("NewVal"=w317:string)  [unwired: 1 in]
        n205 = call <vilib>:"NT Write String.vi"("String"=w317, "Name"="Auto Selector") -> ()  [unwired: 9 in, 1 out]
      }
      event "Command Selection": Value Change {
        # "Get the params and show in table"
        n206 = event-data() -> ("NewVal"=w324:i32)  [unwired: 1 in]
        n207 = property on="Command Selection" class="MCListbox (strict)"() -> ("ItemNames"=w322:string[][])  [unwired: 2 in, 2 out]
        n208 = call <vilib>:"WPI_DashboardUpdate Command Params.vi"("NewVal"=w324, "Commands"=w322, "Param Tbl"=w323) -> ()  [unwired: 8 in, 1 out]
      }
      event "Execute Command": Value Change {
        # "Started one, Unique ID holds\nresponse"
        n209 = event-data() -> ()  [unwired: 1 in, 1 out]
        n210 = property on="Command Selection" class="MCListbox (strict)"() -> ("ItemNames"=w336:string[][])  [unwired: 2 in, 2 out]
        n211 = Index Array(array=w336, index (row)="Command Selection", index (col)=0) -> (element=w334:string)
        n212 = call <vilib>:"Invoke Commands.vi"("Command Params"="Command Params", "Function Name"=w334) -> ("Params"=w330:u8, "Started"=w329:bool)  [unwired: 7 in, 1 out]
        n213 = Array Subset(array="Command Params", length (row)=w330) -> (w331:string[][])  [unwired: 3 in]
        n214 = Select(t="Executing" ("Cmd Status"), s=w329, f="" ("Cmd Status")) -> (s? t:f=→"Cmd Status":string)
      }
      event "Command Selection": Double Click {
        n215 = event-data() -> ("Row"=w346:i32)  [unwired: 1 in]
        n216 = property on="Command Selection" class="MCListbox (strict)"() -> ("ItemNames"=w349:string[][])  [unwired: 2 in, 2 out]
        n217 = local read "Command Params"() -> (w344:string[][])
        n218 = Index Array(array=w349, index (row)=w346, index (col)=0) -> (element=w347:string)
        n219 = call <vilib>:"Invoke Commands.vi"("Command Params"=w344, "Function Name"=w347) -> ("Params"=w343:u8, "Started"=w338:bool)  [unwired: 7 in, 1 out]
        n220 = Array Subset(array=w344, length (row)=w343) -> (w342:string[][])  [unwired: 3 in]
        n221 = Select(t="Executing" ("Cmd Status"), s=w338, f="" ("Cmd Status")) -> (s? t:f=w339:string)
        n222 = local write "Cmd Status"(w339) -> ()
      }
      event "CheckList": Double Click {
        # "Shift clears all"
        # "Update symbols on the listbox"
        n223 = event-data() -> ("PlatMods.Shift"=w352:bool, "Row"=w354:i32)  [unwired: 1 in]
        n224 = case shown="True" w352 {
          tunnel: w354 -> [w358 _]
          tunnel: 1 -> [w357 _]
          frame False {
            n225 = property on="CheckList" class="LstBox (strict)"() -> ("Item Symbols"=w356:i32[])  [unwired: 2 in, 2 out]
            n226 = Replace Array Subset(array=w356, new element=w357, index=w358) -> (w355:i32[])
            n227 = property on="CheckList" class="LstBox (strict)"("Item Symbols"=w355) -> ()  [unwired: 2 in, 2 out]
          }
          frame True {
            w359 = 0 ("Top Row")
            n228 = property on="CheckList" class="LstBox (strict)"() -> ("Number of Rows"=w361:u32)  [unwired: 2 in, 2 out]
            n229 = Initialize Array(0, w361) -> (w360:i32[])
            n230 = property on="CheckList" class="LstBox (strict)"("Top Row"=w359, "Value"=w359, "Item Symbols"=w360) -> ()  [unwired: 2 in, 2 out]
          }
        }
      }
      event "CheckList": Key Down {
        # "Update symbols on the listbox\nLeft and right keys check and uncheck"
        n231 = event-data() -> ("VKey"=w366:T16)  [unwired: 1 in]
        n232 = case shown="\"Left\", \"Right\"" w366 {
          selector: w366 -> [w371 _]
          tunnel: eventvkey."Left" ("VKey") -> [w369 _]
          frame "Left", "Right" {
            n233 = Equal?(x=w369, y=w371) -> (x = y?=w370:bool)
            n234 = Select(t=0, s=w370, f=1) -> (s? t:f=w372:i32)
            n235 = property on="CheckList" class="LstBox (strict)"() -> ("Item Symbols"=w375:i32[])  [unwired: 2 in, 2 out]
            n236 = Replace Array Subset(array=w375, new element=w372, index="CheckList") -> (w374:i32[])
            n237 = property on="CheckList" class="LstBox (strict)"("Item Symbols"=w374) -> ()  [unwired: 2 in, 2 out]
          }
          frame Default {
          }
        }
      }
      event "DB Camera Config": Value Change {
        # "Show or hide the cluster of controls, store in ini file"
        n238 = event-data() -> ("NewVal"=w380:bool)  [unwired: 1 in]
        n239 = case shown="False" w380 {
          tunnel: w379 -> [w389 _]
          tunnel: [w382 w400] -> w378
          tunnel: w377 -> [w381 w400]
          frame False {
            w396 = "Camera"
            w399 = FALSE ("Visible")
            n240 = local read "Camera Settings"() -> (w388:T2)
            n241 = Index Array(array=w389) -> (element=w392:cluster{string[]})  [unwired: 1 in]
            n242 = Unbundle(w388) -> ("Frame Rate"=w387:i32, "Compression"=w386:i32, "Size"=w390:u16)
            n243 = Unbundle(w392) -> (w391:string[])
            n244 = Index Array(array=w391, index=w390) -> (element=w385:string)
            n245 = call-poly <vilib>:"Write Key.vi"("section"=w396, "value"=w385, "key"="Size", "refnum"=w381) -> ("refnum out"=w398:T14)  [unwired: 2 in, 5 out]
            n246 = call-poly <vilib>:"Write Key.vi"("section"=w396, "value"=w387, "key"="FrameRate", "refnum"=w398) -> ("refnum out"=w397:T14)  [unwired: 1 in, 6 out]
            n247 = property on="Camera Settings" class="Clust (strict)"("Visible"=w399) -> ()  [unwired: 2 in, 2 out]
            n248 = local write "DB Camera Config"(w399) -> ()
            n249 = call-poly <vilib>:"Write Key.vi"("section"=w396, "value"=w386, "key"="Compression", "refnum"=w397) -> ("refnum out"=w383:T14)  [unwired: 1 in, 6 out]
            n250 = call <vilib>:"Close Config Data.vi"("refnum"=w383) -> ("file path"=w384:path)  [unwired: 2 in, 8 out]
            n251 = call <vilib>:"Open Config Data.vi"("configuration file path"=w384) -> ("refnum"=w382:T14)  [unwired: 8 in, 2 out]
          }
          frame True {
            n252 = property on="Camera Settings" class="Clust (strict)"("Visible"=TRUE) -> ()  [unwired: 2 in, 2 out]
          }
        }
      }
      event "Camera Settings": Value Change {
        # "Update summary string when any elements of DB camera change"
        n253 = event-data() -> ("NewVal"=w414:T2)  [unwired: 1 in]
        n254 = Index Array(array=w410) -> (element=w409:cluster{string[]})  [unwired: 1 in]
        n255 = Unbundle(w414) -> ("Frame Rate"=w405:i32, "Compression"=w404:i32, "Size"=w407:u16)
        n256 = Unbundle(w409) -> (w408:string[])
        n257 = Index Array(array=w408, index=w407) -> (element=w406:string)
        n258 = Format Into String(format string="%s   %dfps   %d%%", w406, w405, w404) -> (resulting string=w411:string)  [unwired: 2 in, 1 out]
        n259 = Build Array(w411) -> (w412:string[])
        n260 = property on="DB Camera Config" class="Bool (strict)"("Strings [4]"=w412) -> ()  [unwired: 2 in, 2 out]
      }
      event "Motor.Enable": Value Change {
        # "When the test mode otor enable helper is set, update that\ntree row item's value"
        n261 = event-data() -> ("NewVal"=w421:bool)  [unwired: 1 in]
        n262 = Unbundle("Motor") -> ("Value"=w420:dbl)  [unwired: 1 out]
        n263 = Select(t=w420, s=w421, f=0.0) -> (s? t:f=w418:dbl)
        n264 = call <vilib>:"NT Write Number.vi"("Numeric"=w418, "Name"=w417) -> ()  [unwired: 9 in, 1 out]
      }
      event "Test Slider": Value Change {
        # "When the test mode slider helper is set, update that\ntree row item's value"
        n265 = event-data() -> ("NewVal"=w425:dbl)  [unwired: 1 in]
        n266 = call <vilib>:"NT Write Number.vi"("Numeric"=w425, "Name"=w426) -> ()  [unwired: 9 in, 1 out]
      }
      event "On/Off": Value Change {
        # "When the test mode on/off helper value is set, update that\ntree row item's value"
        n267 = event-data() -> ("NewVal"=w431:bool)  [unwired: 1 in]
        n268 = Boolean To (0,1)(Boolean=w431) -> (0, 1=w430:i16)
        n269 = call <vilib>:"NT Write Number.vi"("Numeric"=w430, "Name"=w429) -> ()  [unwired: 9 in, 1 out]
      }
      event "Rev/Fwd": Value Change {
        # "When the test mode helper value for relays is set, update that\ntree row item's value"
        n270 = event-data() -> ("NewVal.Forward"=w440:bool, "NewVal.Reverse"=w439:bool)  [unwired: 1 in]
        n271 = Boolean To (0,1)(Boolean=w440) -> (0, 1=w436:i16)
        n272 = Boolean To (0,1)(Boolean=w439) -> (0, 1=w438:i16)
        n273 = Negate(x=w438) -> (-x=w437:i16)
        n274 = Add(x=w436, y=w437) -> (x+y=w435:i16)
        n275 = call <vilib>:"NT Write Number.vi"("Numeric"=w435, "Name"=w434) -> ()  [unwired: 9 in, 1 out]
      }
      event "Test Ring": Value Change {
        # "When a test mode helper value is selected from the ring,\nset the tree item's variable to the string value"
        n276 = event-data() -> ("NewVal"=w445:u16)  [unwired: 1 in]
        n277 = property on="Test Ring" class="Ring (strict)"() -> ("Strings []"=w446:string[])  [unwired: 2 in, 2 out]
        n278 = Index Array(array=w446, index=w445) -> (element=w444:string)
        n279 = call <vilib>:"NT Write String.vi"("String"=w444, "Name"=w443) -> ()  [unwired: 9 in, 1 out]
      }
      event "Rec Mode": Value Change {
        # "Update globals for recording mode and path to read log from.\nClear when logging and let NetworkTables set path for vision to\nuse."
        n280 = event-data() -> ("NewVal"=w458:enum32{"Stop", "Record", "Playback"})  [unwired: 1 in]
        n281 = global write "WPI_DashboardLogging Global.vi" "Logging Filename"(path "") -> ()
        n282 = global write "WPI_DashboardLogging Global.vi" "Recording"(w458) -> ()
        n283 = case shown="\"Playback\"" w458 {
          tunnel: w457 -> [_ w460 w469]
          tunnel: [_ _ w468] -> w454
          tunnel: [_ _ w467] -> _
          tunnel: w452 -> [_ _ w465]
          tunnel: cluster{i32, i32} {-250, 170} -> [_ _ w464]
          tunnel: [_ _ T17 {"Image Size"=TRUE, "Image Type"=TRUE, "Pixel Value"=TRUE, "ROI Information"=TRUE, "Zoom Factor"=FALSE} ("Image Information Shown:All Elements")] -> w450
          tunnel: [_ _ TRUE ("Zoom Factor")] -> w449
          tunnel: w448 -> [_ _ w461]
          frame Default {
          }
          frame "Stop", "Record" {
            # "Place Window too"
            n284 = invoke class="VI" method="FP.Close"(reference=w460) -> (reference out=w459:refnum<vi>)  [unwired: 2 in, 2 out]
            n285 = invoke class="VI" method="Abort VI"(reference=w459) -> ()  [unwired: 2 in, 3 out]
          }
          frame "Playback" {
            n286 = call "Open Playback Panel.vi"("Offset"=w464, "DB VI Ref"=w465, "Playback in"=w469) -> ("Playback out"=w466:refnum<vi>)  [unwired: 8 in]
            n287 = register-events(w466, w461) -> (reference out=w468:refnum<event-registration>, error out=w467:errorcluster)  [unwired: 2 in]
          }
        }
        n288 = property on="Camera Image" class="ImageControl"("Image Information Shown"=w450, "Image Information Visible"=w449) -> ()  [unwired: 2 in, 2 out]
        n289 = call <vilib>:"WPI_DashboardNT Log FieldName Cache.vi"("Operation"=enum16{"Lookup/Add", "Index", "Clear"}."Clear") -> ()  [unwired: 8 in, 3 out]
      }
      event Panel Close {
        w471 = enum32{"Stop", "Record", "Playback"}."Stop" ("Rec Mode")
        # "Playback window has been closed, abort"
        n290 = event-data() -> ()  [unwired: 1 in, 4 out]
        n291 = local write "Rec Mode"(w471) -> ()
        n292 = global write "WPI_DashboardLogging Global.vi" "Recording"(w471) -> ()
      }
      event Panel Close {
        # "Abort playback window and ourself"
        n293 = event-data() -> ()  [unwired: 1 in, 4 out]
        n294 = invoke class="VI" method="FP.Close"(reference=w477) -> (reference out=w476:refnum<vi>)  [unwired: 2 in, 2 out]
        n295 = invoke class="VI" method="Abort VI"(reference=w476) -> (error out=w475:errorcluster)  [unwired: 2 in, 2 out]
        n296 = invoke class="VI" method="Abort VI"(error in=w475) -> ()  [unwired: 2 in, 3 out]
      }
      event User Event {
        n297 = event-data() -> ("IDs"=w485:cluster{"RPC field ID":u16, "Unique ID":u16}, "String"=w484:string)  [unwired: 1 in]
        n298 = Bundle("IDs"=w485, "String"=w484) -> (w483:T6)  [unwired: 1 in]
        n299 = call <vilib>:"Retrieve RPC Response.vi"("RPC Response"=w483) -> ("Output"=w480:string[][])  [unwired: 10 in]
        n300 = Build Array (concatenate)(w478, w480) -> (w479:string[][])
        n301 = local write "Command Params"(w479) -> ()
        n302 = local write "Cmd Status"("" ("Cmd Status")) -> ()
      }
      event "Vision": Value Change {
        # "Enable/Disable Compression slider.\nHW USB is hard-coded into the camera"
        n303 = event-data() -> ("NewVal"=w492:u16)  [unwired: 1 in]
        n304 = Equal?(x=w492, y=u32 2 ("milliseconds to wait")) -> (x = y?=w490:bool)
        n305 = Select(t=T18."Disabled and Grayed Out" ("Disabled"), s=w490, f=T18."Enabled" ("Disabled")) -> (s? t:f=w487:T18)
        n306 = property on="Compression" class="Slide (strict)"("DisabledEnum"=w487) -> ()  [unwired: 2 in, 2 out]
      }
      event "Tree": Double Click {
        n307 = event-data() -> ("PlatMods"=w497:T21, "Tag"=w496:string)  [unwired: 1 in]
        n308 = Unbundle(w497) -> ("Shift"=w495:bool)  [unwired: 4 out]
        n309 = Not(x=w495) -> (.not. x?=w494:bool)
        n310 = call <vilib>:"NT Update Persistence.vi"("Persistence"=w494, "Name"=w496) -> ()  [unwired: 9 in, 1 out]
      }
    }
  }
  n311 = while {
    tunnel: w49 -> [w501]
    i -> [w504]
    stop <- FALSE stop-if-true
    n312 = Wait (ms)(milliseconds to wait=u32 100) -> ()  [unwired: 1 out]
    n313 = case shown="\"Playback\"" "Rec Mode" {
      tunnel: w504 -> [_ _ w519]
      tunnel: [u32 2829099 ("Base Color") u32 11141120 ("Target Color") w508] -> w500
      frame "Stop", Default {
        # "Reset the color, extra updates don't cost much"
      }
      frame "Record" {
      }
      frame "Playback" {
        # "Playback"
        n314 = Quotient & Remainder(x=w519, y=u32 50 ("milliseconds to wait")) -> (x-y*floor(x/y)=w515:u32)  [unwired: 1 out]
        n315 = Divide(x=w515, y=u32 50 ("milliseconds to wait")) -> (x/y=w512:dbl)
        n316 = Multiply(x=6.283185307179586, y=w512) -> (x*y=w517:dbl)
        n317 = Sine(x=w517) -> (sin(x)=w516:dbl)
        n318 = Absolute Value(x=w516) -> (abs(x)=w509:dbl)
        n319 = call "Interpolate RGB Color.vi"("Proportion"=w509, "Target Color"=u32 30976, "Base Color"=u32 2829099) -> ("Result Color"=w508:u32)  [unwired: 8 in]
      }
    }
    n320 = property class="Pane"(reference=w501, "PaneColor"=w500) -> ()  [unwired: 1 in, 2 out]
  }
  n321 = local write "Dashboard Tab"(T1."Drive" ("Dashboard Tab")) -> ()
  n322 = property on="On/Off" class="Bool (strict)"("Visible"=w17) -> ()  [unwired: 2 in, 2 out]
  n323 = property on="Motor" class="Clust (strict)"("Visible"=w17) -> ()  [unwired: 2 in, 2 out]
  n324 = property on="Progress" class="Clust (strict)"("Visible"=w17) -> ()  [unwired: 2 in, 2 out]
  n325 = property on="Test Ring" class="Ring (strict)"("Visible"=w17) -> ()  [unwired: 2 in, 2 out]
  n326 = property on="Rev/Fwd" class="Clust (strict)"("Visible"=w17) -> ()  [unwired: 2 in, 2 out]
  n327 = property on="Camera Settings" class="Clust (strict)"("Visible"=w17) -> ()  [unwired: 2 in, 2 out]
  n328 = while {
    tunnel: u16 1741 ("timeout ms (25000)") -> [w521]
    stop <- FALSE stop-if-true
    n329 = TCP Create Listener(10:w521) -> (0:w520:errorcluster, 3:w522:refnum<k5>)  [unwired: 4 in, 1 out]
    n330 = case shown="No Error" w520 {
      selector: w520 -> [w524 _]
      tunnel: w522 -> [w525 _]
      frame No Error {
        n331 = while {
          tunnel: w525 -> [w528]
          tunnel: w524 -> [w527]
          stop <- FALSE stop-if-true
          n332 = TCP Wait On Listener(8:w527, 11:w528) -> (0:w529:errorcluster, 4:w530:refnum<k5>)  [unwired: 2 in, 3 out]
          n333 = local write "TCP"(w530) -> ()
          n334 = case shown="No Error" w529 {
            frame No Error {
            }
            frame Error {
              n335 = Wait (ms)(milliseconds to wait=u32 1000) -> ()  [unwired: 1 out]
            }
          }
        }
      }
      frame Error {
        n336 = Wait (ms)(milliseconds to wait=u32 1000) -> ()  [unwired: 1 out]
      }
    }
  }
  n337 = local write "DB Camera Config"(w17) -> ()
  n338 = local write "Command Params"(string[][] [] ("Command Params")) -> ()
  n339 = global write "WPI_DashboardLogging Global.vi" "Recording"(w43) -> ()
  n340 = local write "Command Selection"(u16 0 ("milliseconds to wait")) -> ()
  n341 = local write "Rec Mode"(w43) -> ()
  n342 = call-poly <vilib>:"NT Write Value.vi"("String"="Auto", "Name"="Auto Selector") -> ()  [unwired: 9 in, 1 out]
